vi "LINC Register COSMOS File.vi"(6 "scaling (T)":bool=TRUE, 8 "error in (no error)":errorcluster, 9 "target name override":string, 10 "path":path=path "C:/Projects/LabVIEW 8.5.1 Programs/Common Components/LINC/Examples/APP_TLM.txt", 11 "LINC session":refnum<class "LINC.lvclass">) -> (0 "error out":errorcluster, 3 "dup LINC session":refnum<class "LINC.lvclass">)   [LabVIEW 2018, in "STEPkgDriver_LINC.lvlib" / "LINC.lvclass"]
uses:
  LINC.lvclass
  LINC Format Prototype.ctl
  STEPkgDriver_LINC.lvlib
  LINC Packet.ctl
  LINC Packet Fields.ctl
  LINC Macro.ctl
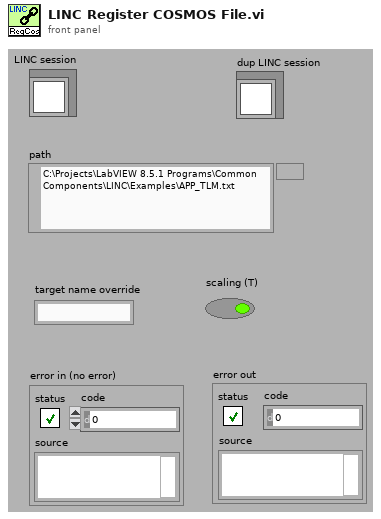
[diagram p1: front panel]
types:
  T1 = typedef "STEPkgDriver_LINC.lvlib/LINC Packet.ctl" = cluster{"type":enum16{"CMD", "TLM"}, "description":string, "hazardous":bool, "item names":string[], "item formats":T2[]}
  T2 = typedef "STEPkgDriver_LINC.lvlib/LINC Format Prototype.ctl" = cluster{"type":string, "bit offset":i32, "bit size":i32, "format":string, "unit":string, "description":string, "state values":i64[], "states":string[], "max":string, "min":string, "default":string, "array":bool, "bit element size":i32, "poly bound":dbl[], "poly scale":cluster{"coefficients":dbl[]}[], "labview size":i32, "simulate":bool, "ID":bool, "required":bool}
  T3 = typedef "STEPkgDriver_LINC.lvlib/LINC Macro.ctl" = cluster{"enabled":bool, "start":i32, "length":i32, "format":string}
  T4 = enum16{"Default", "COMMAND", "SELECT_COMMAND", "HIDDEN", "DISABLED", "DISABLE_MESSAGES", "META", "HAZARDOUS", "PARAMETER", "APPEND_PARAMETER", "ID_PARAMETER", "APPEND_ID_PARAMETER", "ARRAY_PARAMETER", "APPEND_ARRAY_PARAMETER", "SELECT_PARAMETER", "MACRO_APPEND_START", "MACRO_APPEND_END", "PROCESSOR", "ALLOW_SHORT", "STATE", "REQUIRED", "WRITE_CONVERSION", "READ_CONVERSION", "POLY_WRITE_CONVERSION", "POLY_READ_CONVERSION", "SEG_POLY_WRITE_CONVERSION", "SEG_POLY_READ_CONVERSION", "GENERIC_WRITE_CONVERSION_START", "GENERIC_WRITE_CONVERSION_END", "GENERIC_READ_CONVERSION_START", "GENERIC_READ_CONVERSION_END", "FORMAT_STRING ", "MINIMUM_VALUE", "MAXIMUM_VALUE", "DEFAULT_VALUE", "DESCRIPTION", "TELEMETRY", "SELECT_TELEMETRY", "LIMITS_GROUP", "LIMITS_GROUP_ITEM", "ITEM", "APPEND_ITEM", "ID_ITEM", "APPEND_ID_ITEM", "ARRAY_ITEM", "APPEND_ARRAY_ITEM", "LIMITS", "LIMITS_RESPONSE", "UNITS", "SELECT_ITEM"}
  T5 = typedef "STEPkgDriver_LINC.lvlib/LINC Packet Fields.ctl" = cluster{"name":string, "bit offset":string, "bit size":string, "type":string, "min":string, "max":string, "default":string, "description":string, "total size":string}
  T6 = enum16{"state", "required", "poly scale", "format string", "minimum value", "maximum value", "default value", "description", "units"}
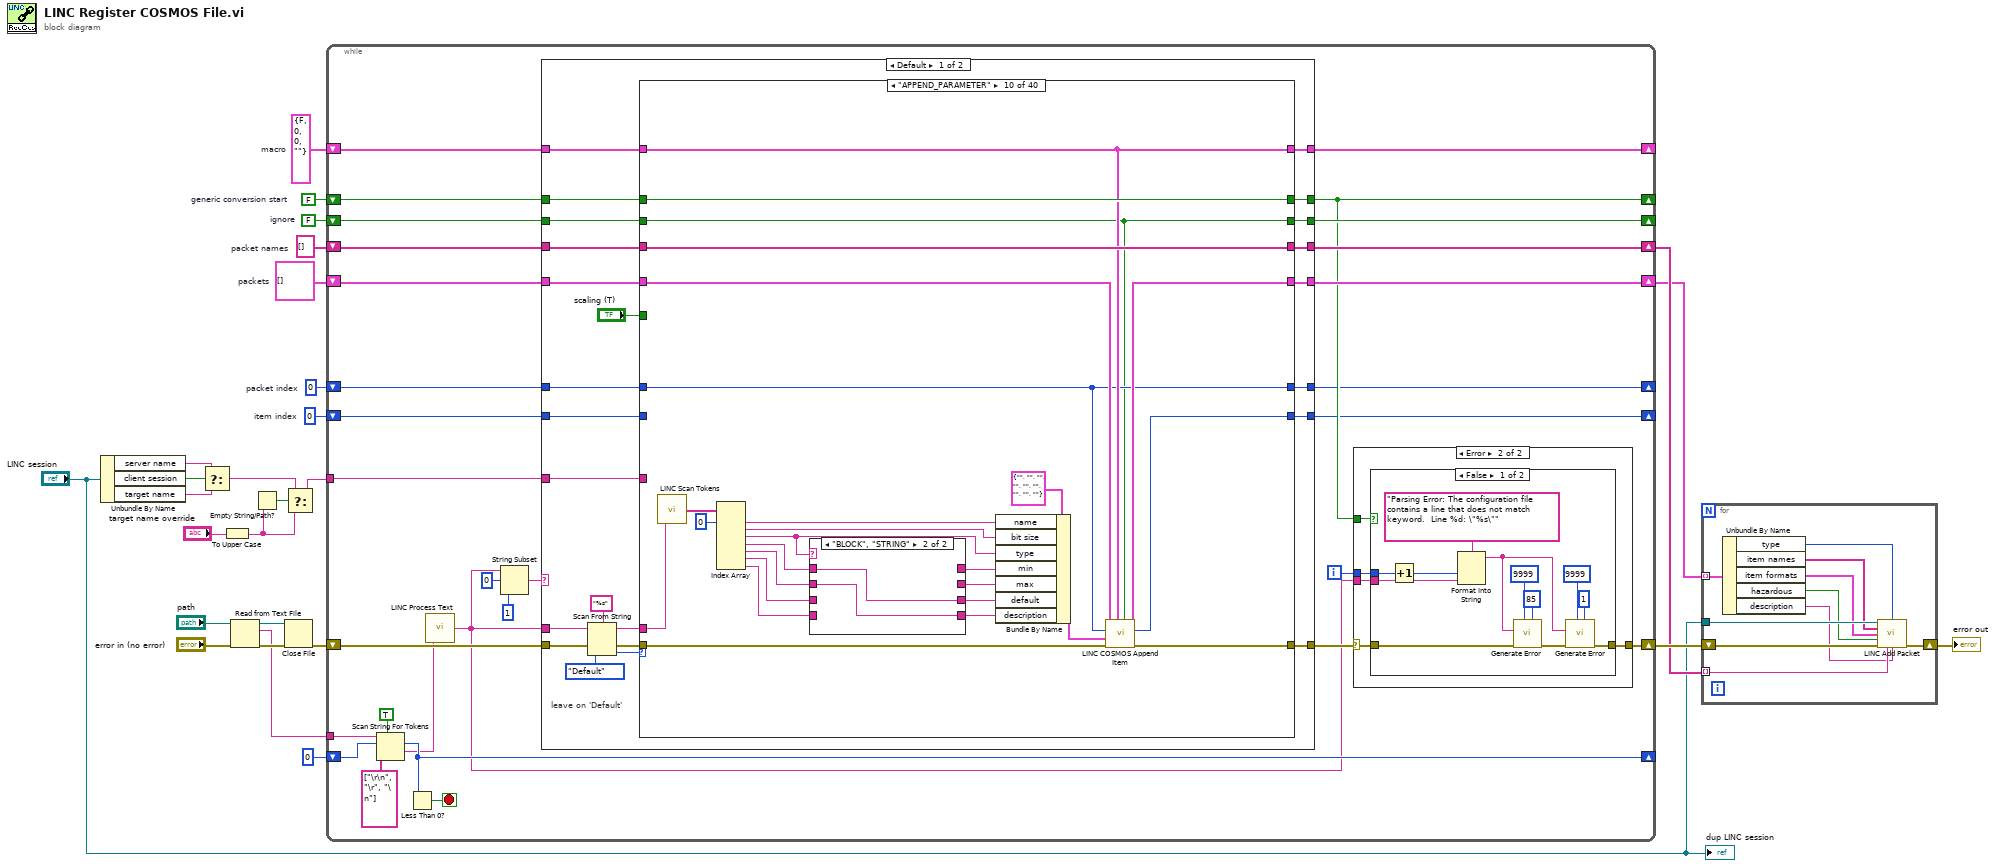
[diagram p0: block diagram]
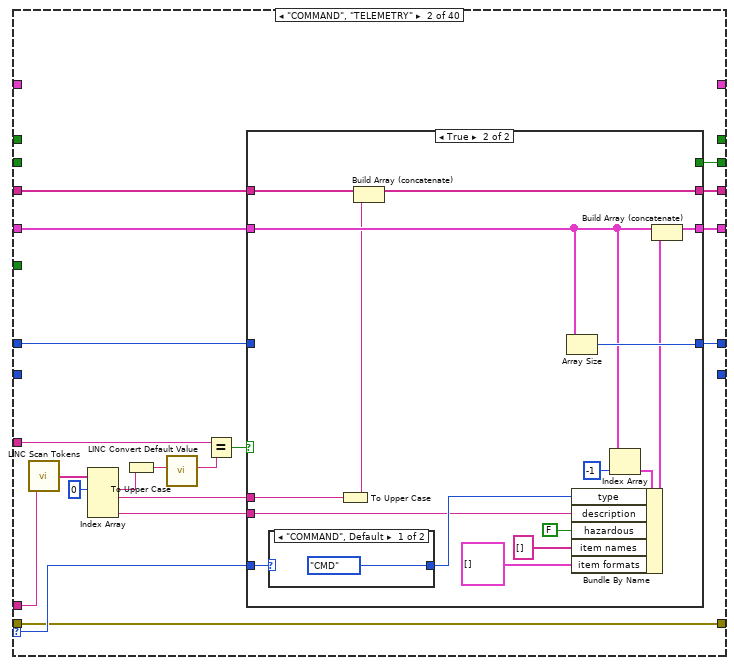
[diagram p5: hidden frame]
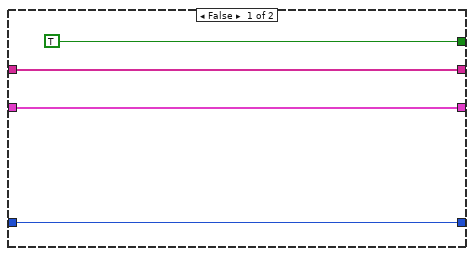
[diagram p6: hidden frame]
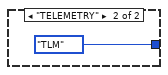
[diagram p7: hidden frame]
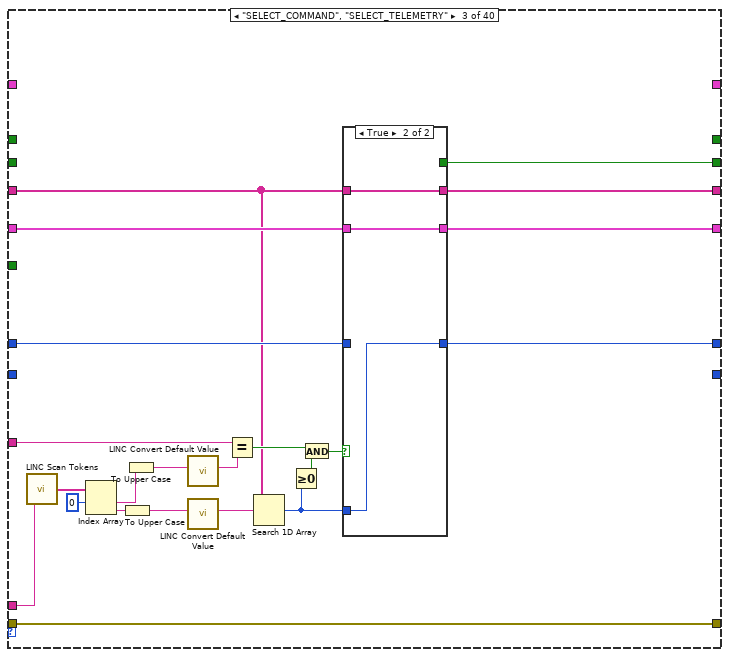
[diagram p8: hidden frame]
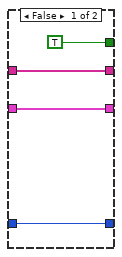
[diagram p9: hidden frame]
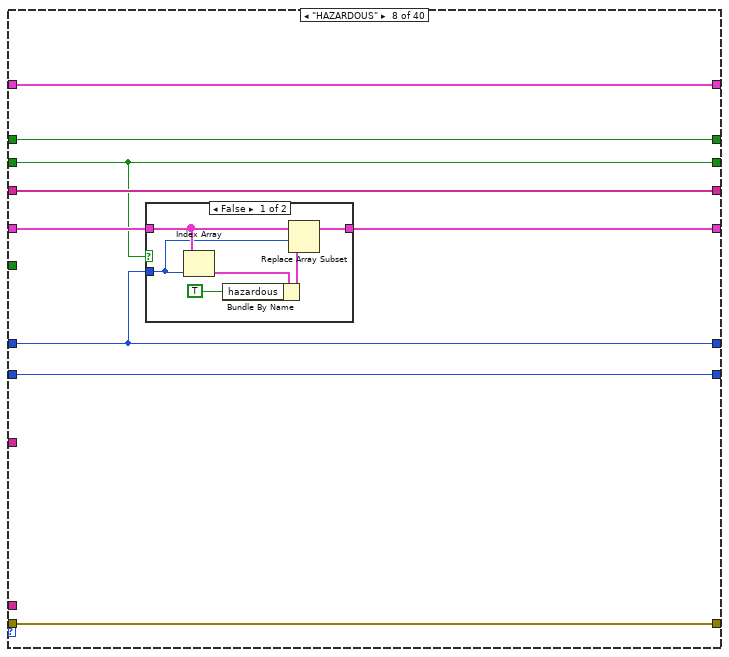
[diagram p14: hidden frame]
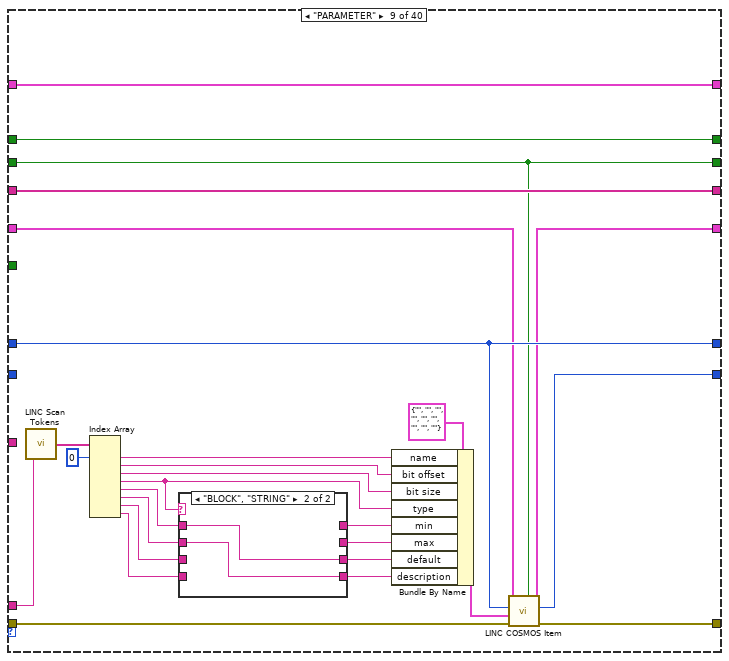
[diagram p16: hidden frame]
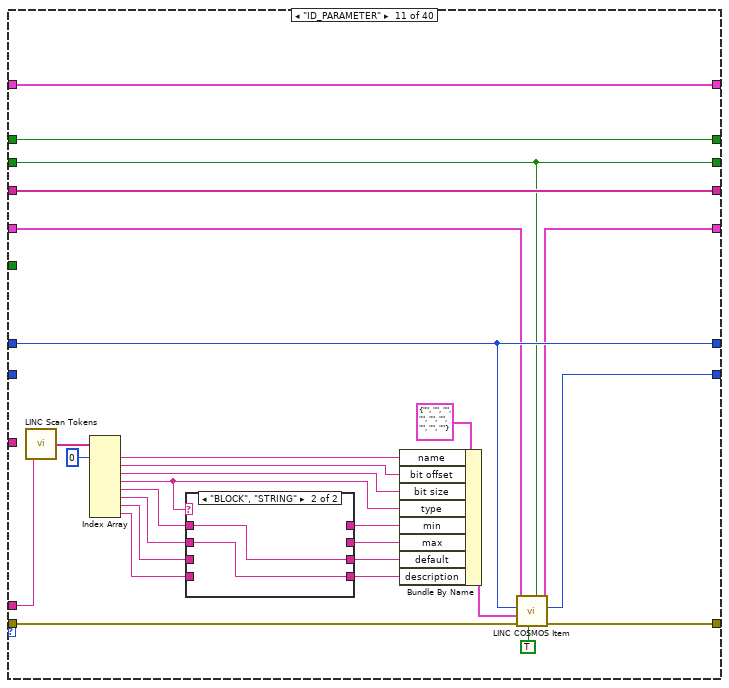
[diagram p19: hidden frame]
diagram:
  w14 = T1[] []  # packets
  w15 = T3 {"enabled"=FALSE, "start"=0, "length"=0, "format"=""}  # macro
  w16 = string[] []  # packet names
  w17 = 0  # item index
  w18 = 0  # packet index
  w19 = FALSE  # generic conversion start
  w22 = FALSE  # ignore
  n1 = Unbundle By Name("LINC session") -> ("server name"=w8:string, "client session"=w9:bool, "target name"=w7:string)
  n2 = Select(t=w8, s=w9, f=w7) -> (s? t:f=w4:string)
  n3 = To Upper Case(1:"target name override") -> (0:w1:string)
  n4 = Read from Text File(file (use dialog)="path", error in="error in (no error)") -> (refnum out=w25:refnum<file>, text=w23:string, error out=w26:errorcluster)  [unwired: 2 in, 1 out]
  n5 = Empty String/Path?(string/path=w1) -> (empty?=w5:bool)
  n6 = Close File(refnum=w25, error in=w26) -> (error out=w21:errorcluster)  [unwired: 1 out]
  n7 = Select(t=w4, s=w5, f=w1) -> (s? t:f=w3:string)
  n8 = while {
    tunnel: w23 -> [w57]
    shift-right: [w53] -> _
    shift-left: 0 -> [w56]
    shift-right: [w37] -> w13
    shift-left: w21 -> [w51]
    shift-right: [w48] -> _
    shift-left: w22 -> [w49]
    shift-right: [w45] -> w11
    shift-left: w16 -> [w47]
    shift-right: [w44] -> w10
    shift-left: w14 -> [w46]
    shift-right: [w39] -> _
    shift-left: w19 -> [w40]
    shift-right: [w32] -> _
    shift-left: w18 -> [w34]
    shift-right: [w31] -> _
    shift-left: w17 -> [w33]
    shift-right: [w29] -> _
    shift-left: w15 -> [w30]
    tunnel: w3 -> [w28]
    i -> [w36]
    stop <- w52 stop-if-true
    n9 = Scan String For Tokens(5:TRUE ("allow empty tokens? (F)"), 6:string[] ["\r\n", "\r", "\n"] ("delimiters (\\s,\\t,\\r,\\n)"), 8:w56, 9:w57) -> (1:w50:string, 2:w53:i32)  [unwired: 2 in, 2 out]
    n10 = Less Than 0?(x=w53) -> (x < 0?=w52:bool)
    n11 = call "LINC Process Text.vi"("line in"=w50) -> ("line out"=w35:string)
    n12 = String Subset(string=w35, offset (0)=0, length (rest)=1 ("length (rest)")) -> (substring=w41:string)
    n13 = case shown="Default" w41 {
      tunnel: w51 -> [w99 w850]
      tunnel: [w93 w850] -> w38
      tunnel: w35 -> [w97 _]
      tunnel: w49 -> [w92 w849]
      tunnel: [w91 w849] -> w48
      tunnel: w47 -> [w90 w848]
      tunnel: w46 -> [w89 w847]
      tunnel: [w88 w848] -> w45
      tunnel: [w87 w847] -> w44
      tunnel: w40 -> [w86 w846]
      tunnel: [w85 w846] -> w39
      tunnel: w34 -> [w84 w845]
      tunnel: w33 -> [w83 w844]
      tunnel: [w82 w845] -> w32
      tunnel: [w81 w844] -> w31
      tunnel: w30 -> [w80 w843]
      tunnel: [w79 w843] -> w29
      tunnel: w28 -> [w77 _]
      frame Default {
        # "leave on 'Default'"
        n14 = Scan From String(format string="%s", input string=w97, error in=w99, default 1=T4."Default") -> (remaining string=w94:string, error out=w96:errorcluster, output 1=w95:T4)  [unwired: 1 in, 1 out]
        n15 = case shown="\"APPEND_PARAMETER\"" w95 {
          selector: w95 -> [_ w125 _ _ _ _ _ _ _ _ _ _ _ _ _ _ _ _ _ _ _ _ _ _ _ _ _ _ _ _ _ _ _ _ _ _ _ _ _ _]
          tunnel: w96 -> [w103 w120 w170 w182 w190 w198 w206 w217 w246 w279 w312 w346 w373 w394 w408 w429 w444 w449 w457 w477 w493 w500 w521 w571 w609 w617 w630 w648 w666 w684 w702 w715 w723 w745 w760 w786 w803 w813 w821 w834]
          tunnel: w94 -> [_ w122 w166 _ _ _ _ _ w249 w280 w315 w347 w375 w396 w403 w430 _ _ _ w484 _ _ w513 w563 _ _ w634 w652 w670 w688 w706 _ _ w732 w761 w772 w804 _ _ w838]
          tunnel: [w103 w120 w170 w182 w190 w198 w206 w217 w245 w278 w311 w345 w372 w393 w408 w429 w444 w449 w457 w476 w492 w500 w520 w570 w609 w617 w629 w647 w665 w683 w701 w715 w723 w744 w759 w785 w802 w813 w821 w833] -> w93
          tunnel: w92 -> [w107 _ _ w185 w193 w201 w209 w210 w235 w268 w300 w334 w358 w379 w410 w423 w442 w452 w460 w463 w485 w503 w514 w564 w612 w620 w623 w641 w659 w677 w695 w718 w726 w729 w747 w768 w790 w816 w824 w827]
          tunnel: [w107 w126 w150 w185 w193 w201 w209 w210 w235 w268 w300 w334 w358 w379 w410 w423 w442 w452 w460 w463 w485 w503 w508 w558 w612 w620 w623 w641 w659 w677 w695 w718 w726 w729 w747 w768 w790 w816 w824 w827] -> w91
          tunnel: w90 -> [w106 w115 w153 w184 w192 w200 w208 w218 w248 w283 w314 w350 w369 w390 w406 w422 w441 w451 w459 w480 w495 w502 w507 w557 w611 w619 w638 w656 w674 w692 w710 w717 w725 w740 w764 w781 w807 w815 w823 w842]
          tunnel: w89 -> [w105 w117 w154 w183 w191 w199 w207 w213 w238 w277 w304 w344 w371 w392 w409 w421 w440 w450 w458 w482 w491 w501 w517 w567 w610 w618 w628 w646 w664 w682 w700 w716 w724 w743 w758 w784 w801 w814 w822 w832]
          tunnel: [w106 w114 w152 w184 w192 w200 w208 w218 w248 w283 w314 w350 w369 w390 w406 w422 w441 w451 w459 w480 w495 w502 w506 w556 w611 w619 w638 w656 w674 w692 w710 w717 w725 w740 w764 w781 w807 w815 w823 w842] -> w88
          tunnel: [w105 w116 w151 w183 w191 w199 w207 w212 w237 w276 w303 w343 w370 w391 w409 w421 w440 w450 w458 w483 w490 w501 w516 w566 w610 w618 w627 w645 w663 w681 w699 w716 w724 w742 w757 w783 w800 w814 w822 w831] -> w87
          tunnel: w86 -> [w104 _ _ w181 w189 w197 w205 w216 w252 w284 w318 w351 w378 w398 w407 w424 w443 w448 w456 w481 w494 w499 w510 w560 _ _ w637 w655 w673 w691 w709 w714 w722 w746 w765 w787 w808 w812 w820 w841]
          tunnel: [w104 _ _ w181 w189 w197 w205 w216 w252 w284 w318 w351 w378 w398 w407 w424 w443 w448 w456 w481 w494 w499 w509 w559 TRUE FALSE w637 w655 w673 w691 w709 w714 w722 w746 w765 w787 w808 w812 w820 w841] -> w85
          tunnel: w84 -> [w102 w108 w156 w179 w187 w195 w203 w211 w239 w269 w305 w335 w368 w389 w400 w420 w439 w446 w454 w479 w488 w497 w519 w569 w607 w615 w626 w644 w662 w680 w698 w712 w720 w730 w749 w769 w792 w810 w818 w830]
          tunnel: w83 -> [w101 _ _ w178 w186 w194 w202 w214 _ _ _ _ _ _ _ w419 w438 w445 w453 w478 w487 w496 w518 w568 w606 w614 w625 w643 w661 w679 w697 w711 w719 _ _ _ _ w809 w817 w829]
          tunnel: [w102 w119 w155 w179 w187 w195 w203 w211 w239 w269 w305 w335 w368 w389 w400 w420 w439 w446 w454 w479 w488 w497 w505 w555 w607 w615 w626 w644 w662 w680 w698 w712 w720 w730 w749 w769 w792 w810 w818 w830] -> w82
          tunnel: [w101 _ _ w178 w186 w194 w202 w214 w236 w275 w302 w342 w367 w388 w399 w419 w438 w445 w453 w478 w487 w496 w504 w554 w606 w614 w625 w643 w661 w679 w697 w711 w719 w739 w756 w780 w799 w809 w817 w829] -> w81
          tunnel: w80 -> [w100 _ _ w180 w188 w196 w204 w215 w247 w270 w313 w337 w374 w395 w401 w426 w437 w447 w455 w475 w489 w498 w515 w565 w608 w616 w624 w642 w660 w678 w696 w713 w721 w741 w750 w782 w793 w811 w819 w828]
          tunnel: [w100 _ _ w180 w188 w196 w204 w215 w247 w270 w313 w337 w374 w395 w401 w425 w436 w447 w455 w475 w489 w498 w511 w561 w608 w616 w624 w642 w660 w678 w696 w713 w721 w741 w750 w782 w793 w811 w819 w828] -> w79
          tunnel: w77 -> [_ w110 w160 _ _ _ _ _ _ _ _ _ _ _ _ _ _ _ _ _ _ _ _ _ _ _ _ _ _ _ _ _ _ _ _ _ _ _ _ _]
          tunnel: "scaling (T)" -> [_ _ _ _ _ _ _ _ _ _ _ _ _ _ _ _ _ _ _ _ _ _ w512 w562 _ _ _ _ _ _ _ _ _ _ _ _ _ _ _ _]
          frame "Default" {
          }
          frame "COMMAND", "TELEMETRY" {
            n16 = call "LINC Scan Tokens.vi"("string"=w122) -> ("tokens"=w124:string[])
            n17 = Index Array(array=w124, index #1=0 ("index")) -> (element #1=w113:string, element #2=w121:string, element #4=w118:string)  [unwired: 3 in, 1 out]
            n18 = To Upper Case(1:w113) -> (0:w112:string)
            n19 = call "LINC Convert Default Value.vi"("default in"=w112) -> ("default out"=w111:string)  [unwired: 10 in]
            n20 = Equal?(x=w110, y=w111) -> (x = y?=w109:bool)
            n21 = case shown="True" w109 {
              tunnel: [TRUE _] -> w126
              tunnel: w125 -> [_ w146]
              tunnel: w121 -> [_ w145]
              tunnel: [w127 w144] -> w119
              tunnel: w118 -> [_ w140]
              tunnel: w117 -> [w128 w136]
              tunnel: [w128 w135] -> w116
              tunnel: w115 -> [w129 w133]
              tunnel: [w129 w132] -> w114
              tunnel: w108 -> [w127 _]
              frame False {
              }
              frame True {
                n22 = case shown="\"COMMAND\", Default" w146 {
                  tunnel: [enum16{"CMD", "TLM"}."CMD" enum16{"CMD", "TLM"}."TLM"] -> w141
                  frame "COMMAND", Default {
                  }
                  frame "TELEMETRY" {
                  }
                }
                n23 = To Upper Case(1:w145) -> (0:w131:string)
                n24 = Build Array (concatenate)(w133, w131) -> (w132:string[])
                n25 = Array Size(array=w136) -> (size(s)=w144:i32)
                n26 = Index Array(array=w136, index=-1) -> (element=w142:T1)
                n27 = Bundle By Name(cluster=w142, "type"=w141, "description"=w140, "hazardous"=FALSE, "item names"=string[] [], "item formats"=T2[] []) -> (w134:T1)
                n28 = Build Array (concatenate)(w136, w134) -> (w135:T1[])
              }
            }
          }
          frame "SELECT_COMMAND", "SELECT_TELEMETRY" {
            n29 = call "LINC Scan Tokens.vi"("string"=w166) -> ("tokens"=w169:string[])
            n30 = Index Array(array=w169, index #1=0 ("index")) -> (element #1=w163:string, element #2=w167:string)  [unwired: 1 in]
            n31 = To Upper Case(1:w167) -> (0:w162:string)
            n32 = To Upper Case(1:w163) -> (0:w165:string)
            n33 = call "LINC Convert Default Value.vi"("default in"=w165) -> ("default out"=w164:string)  [unwired: 10 in]
            n34 = call "LINC Convert Default Value.vi"("default in"=w162) -> ("default out"=w161:string)  [unwired: 10 in]
            n35 = Equal?(x=w160, y=w164) -> (x = y?=w159:bool)
            n36 = Search 1D Array(1D array=w153, element=w161) -> (index of element=w149:i32)  [unwired: 1 in]
            n37 = Greater Or Equal To 0?(x=w149) -> (x >= 0?=w158:bool)
            n38 = And(x=w159, y=w158) -> (x .and. y?=w157:bool)
            n39 = case shown="True" w157 {
              tunnel: w156 -> [w171 _]
              tunnel: w149 -> [_ w177]
              tunnel: [w171 w177] -> w155
              tunnel: w154 -> [w172 w175]
              tunnel: w153 -> [w173 w176]
              tunnel: [w173 w176] -> w152
              tunnel: [w172 w175] -> w151
              tunnel: [TRUE _] -> w150
              frame False {
              }
              frame True {
              }
            }
          }
          frame "HIDDEN" {
            # "Ignore"
          }
          frame "DISABLED" {
            # "Ignore"
          }
          frame "DISABLE_MESSAGES" {
            # "Ignore"
          }
          frame "META" {
            # "Ignore"
          }
          frame "HAZARDOUS" {
            n40 = case shown="False" w210 {
              tunnel: w213 -> [w222 w225]
              tunnel: [w221 w225] -> w212
              tunnel: w211 -> [w220 _]
              frame False {
                n41 = Index Array(array=w222, index=w220) -> (element=w224:T1)
                n42 = Bundle By Name(cluster=w224, "hazardous"=TRUE) -> (w223:T1)
                n43 = Replace Array Subset(array=w222, new element=w223, index=w220) -> (w221:T1[])
              }
              frame True {
              }
            }
          }
          frame "PARAMETER" {
            n44 = call "LINC Scan Tokens.vi"("string"=w249) -> ("tokens"=w251:string[])
            n45 = Index Array(array=w251, index #1=0 ("index")) -> (element #1=w243:string, element #2=w242:string, element #3=w241:string, element #4=w234:string, element #5=w233:string, element #6=w232:string, element #7=w231:string, element #8=w230:string)  [unwired: 7 in]
            n46 = case shown="\"BLOCK\", \"STRING\"" w234 {
              tunnel: [w256 _] -> w229
              tunnel: [w255 _] -> w228
              tunnel: [w254 w258] -> w227
              tunnel: w233 -> [w256 w258]
              tunnel: w232 -> [w255 w257]
              tunnel: w231 -> [w254 _]
              tunnel: w230 -> [w253 _]
              tunnel: [w253 w257] -> w226
              frame Default {
              }
              frame "BLOCK", "STRING" {
              }
            }
            n47 = Bundle By Name(cluster=T5 {"name"="", "bit offset"="", "bit size"="", "type"="", "min"="", "max"="", "default"="", "description"="", "total size"=""} ("packet fields"), "name"=w243, "bit offset"=w242, "bit size"=w241, "type"=w234, "min"=w229, "max"=w228, "default"=w227, "description"=w226) -> (w240:T5)
            n48 = call "LINC COSMOS Item.vi"("ignore"=w235, "error in (no error)"=w246, "packet fields"=w240, "packet index"=w239, "packets in"=w238) -> ("error out"=w245:errorcluster, "item index"=w236:i32, "packets out"=w237:T1[])  [unwired: 4 in]
          }
          frame "APPEND_PARAMETER" {
            n49 = call "LINC Scan Tokens.vi"("string"=w280) -> ("tokens"=w281:string[])
            n50 = Index Array(array=w281, index #1=0 ("index")) -> (element #1=w273:string, element #2=w272:string, element #3=w263:string, element #4=w262:string, element #5=w261:string, element #6=w260:string, element #7=w259:string)  [unwired: 6 in]
            n51 = case shown="\"BLOCK\", \"STRING\"" w263 {
              tunnel: [w288 _] -> w267
              tunnel: [w287 _] -> w266
              tunnel: [w286 w290] -> w265
              tunnel: w262 -> [w288 w290]
              tunnel: w261 -> [w287 w289]
              tunnel: w260 -> [w286 _]
              tunnel: w259 -> [w285 _]
              tunnel: [w285 w289] -> w264
              frame Default {
              }
              frame "BLOCK", "STRING" {
              }
            }
            n52 = Bundle By Name(cluster=T5 {"name"="", "bit offset"="", "bit size"="", "type"="", "min"="", "max"="", "default"="", "description"="", "total size"=""} ("packet fields"), "name"=w273, "bit size"=w272, "type"=w263, "min"=w267, "max"=w266, "default"=w265, "description"=w264) -> (w271:T5)
            n53 = call "LINC COSMOS Append Item.vi"("ignore"=w268, "macro"=w270, "error in (no error)"=w279, "packet fields"=w271, "packet index"=w269, "packets in"=w277) -> ("error out"=w278:errorcluster, "item index"=w275:i32, "packets out"=w276:T1[])  [unwired: 3 in]
          }
          frame "ID_PARAMETER" {
            n54 = call "LINC Scan Tokens.vi"("string"=w315) -> ("tokens"=w317:string[])
            n55 = Index Array(array=w317, index #1=0 ("index")) -> (element #1=w309:string, element #2=w308:string, element #3=w307:string, element #4=w295:string, element #5=w294:string, element #6=w293:string, element #7=w292:string, element #8=w291:string)  [unwired: 7 in]
            n56 = case shown="\"BLOCK\", \"STRING\"" w295 {
              tunnel: [w322 _] -> w299
              tunnel: [w321 _] -> w298
              tunnel: [w320 w324] -> w297
              tunnel: w294 -> [w322 w324]
              tunnel: w293 -> [w321 w323]
              tunnel: w292 -> [w320 _]
              tunnel: w291 -> [w319 _]
              tunnel: [w319 w323] -> w296
              frame Default {
              }
              frame "BLOCK", "STRING" {
              }
            }
            n57 = Bundle By Name(cluster=T5 {"name"="", "bit offset"="", "bit size"="", "type"="", "min"="", "max"="", "default"="", "description"="", "total size"=""} ("packet fields"), "name"=w309, "bit offset"=w308, "bit size"=w307, "type"=w295, "min"=w299, "max"=w298, "default"=w297, "description"=w296) -> (w306:T5)
            n58 = call "LINC COSMOS Item.vi"("ignore"=w300, "ID?"=TRUE, "error in (no error)"=w312, "packet fields"=w306, "packet index"=w305, "packets in"=w304) -> ("error out"=w311:errorcluster, "item index"=w302:i32, "packets out"=w303:T1[])  [unwired: 3 in]
          }
          frame "APPEND_ID_PARAMETER" {
            n59 = call "LINC Scan Tokens.vi"("string"=w347) -> ("tokens"=w348:string[])
            n60 = Index Array(array=w348, index #1=0 ("index")) -> (element #1=w340:string, element #2=w339:string, element #3=w332:string, element #4=w328:string, element #5=w327:string, element #6=w326:string, element #7=w325:string)  [unwired: 6 in]
            n61 = case shown="\"BLOCK\", \"STRING\"" w332 {
              tunnel: [w355 _] -> w333
              tunnel: [w354 _] -> w331
              tunnel: [w353 w357] -> w330
              tunnel: w328 -> [w355 w357]
              tunnel: w327 -> [w354 w356]
              tunnel: w326 -> [w353 _]
              tunnel: w325 -> [w352 _]
              tunnel: [w352 w356] -> w329
              frame Default {
              }
              frame "BLOCK", "STRING" {
              }
            }
            n62 = Bundle By Name(cluster=T5 {"name"="", "bit offset"="", "bit size"="", "type"="", "min"="", "max"="", "default"="", "description"="", "total size"=""} ("packet fields"), "name"=w340, "bit size"=w339, "type"=w332, "min"=w333, "max"=w331, "default"=w330, "description"=w329) -> (w338:T5)
            n63 = call "LINC COSMOS Append Item.vi"("ignore"=w334, "ID?"=TRUE, "macro"=w337, "error in (no error)"=w346, "packet fields"=w338, "packet index"=w335, "packets in"=w344) -> ("error out"=w345:errorcluster, "item index"=w342:i32, "packets out"=w343:T1[])  [unwired: 2 in]
          }
          frame "ARRAY_PARAMETER", "ARRAY_ITEM" {
            n64 = call "LINC Scan Tokens.vi"("string"=w375) -> ("tokens"=w377:string[])
            n65 = Index Array(array=w377, index #1=0 ("index")) -> (element #1=w365:string, element #2=w364:string, element #3=w363:string, element #4=w362:string, element #5=w360:string, element #6=w359:string)  [unwired: 5 in]
            n66 = Bundle By Name(cluster=T5 {"name"="", "bit offset"="", "bit size"="", "type"="", "min"="", "max"="", "default"="", "description"="", "total size"=""} ("packet fields"), "name"=w365, "bit offset"=w364, "bit size"=w363, "type"=w362, "total size"=w360, "description"=w359) -> (w361:T5)
            n67 = call "LINC COSMOS Array Item.vi"("ignore"=w358, "error in (no error)"=w373, "packet fields"=w361, "packet index"=w368, "packets in"=w371) -> ("error out"=w372:errorcluster, "item index"=w367:i32, "packets out"=w370:T1[])  [unwired: 4 in]
          }
          frame "APPEND_ARRAY_PARAMETER", "APPEND_ARRAY_ITEM" {
            n68 = call "LINC Scan Tokens.vi"("string"=w396) -> ("tokens"=w397:string[])
            n69 = Index Array(array=w397, index #1=0 ("index")) -> (element #1=w381:string, element #2=w386:string, element #3=w385:string, element #4=w383:string, element #5=w382:string)  [unwired: 4 in]
            n70 = Bundle By Name(cluster=T5 {"name"="", "bit offset"="", "bit size"="", "type"="", "min"="", "max"="", "default"="", "description"="", "total size"=""} ("packet fields"), "name"=w381, "bit size"=w386, "type"=w385, "total size"=w383, "description"=w382) -> (w384:T5)
            n71 = call "LINC COSMOS Append Array Item.vi"("ignore"=w379, "error in (no error)"=w394, "packet fields"=w384, "packet index"=w389, "packets in"=w392) -> ("error out"=w393:errorcluster, "item index"=w388:i32, "packets out"=w391:T1[])  [unwired: 4 in]
          }
          frame "SELECT_PARAMETER", "SELECT_ITEM" {
            n72 = call "LINC Scan Tokens.vi"("string"=w403) -> ("tokens"=w405:string[])
            n73 = Index Array(array=w405, index=0) -> (element=w402:string)
            n74 = Search 1D Array(1D array=w406, element=w402) -> (index of element=w399:i32)  [unwired: 1 in]
          }
          frame "MACRO_APPEND_START" {
            n75 = call "LINC Scan Tokens.vi"("string"=w430) -> ("tokens"=w432:string[])
            n76 = Index Array(array=w432, index #1=0 ("index")) -> (element #1=w428:string, element #2=w427:string, element #3=w413:string)  [unwired: 2 in]
            n77 = Empty String/Path?(string/path=w413) -> (empty?=w414:bool)
            n78 = case shown="True" w414 {
              tunnel: w413 -> [w433 _]
              tunnel: [w433 "%s%d"] -> w412
              frame False {
              }
              frame True {
              }
            }
            n79 = Decimal String To Number(string=w428) -> (number=w417:i32)  [unwired: 2 in, 1 out]
            n80 = Decimal String To Number(string=w427) -> (number=w418:i32)  [unwired: 2 in, 1 out]
            n81 = Subtract(x=w418, y=w417) -> (x-y=w416:i32)
            n82 = Increment(x=w416) -> (x+1=w415:i32)
            n83 = Bundle By Name(cluster=w426, "enabled"=TRUE, "start"=w417, "length"=w415, "format"=w412) -> (w425:T3)
          }
          frame "MACRO_APPEND_END" {
            n84 = Bundle By Name(cluster=w437, "enabled"=FALSE) -> (w436:T3)
          }
          frame "PROCESSOR" {
            # "Ignore"
          }
          frame "ALLOW_SHORT" {
            # "Ignore"
          }
          frame "STATE" {
            n85 = call "LINC Scan Tokens.vi"("string"=w484) -> ("tokens"=w473:string[])
            n86 = Index Array(array=w473, index #1=0 ("index")) -> (element #1=w471:string, element #2=w472:string)  [unwired: 1 in]
            n87 = Decimal String To Number(string=w472, default (0L)=i64 0) -> (number=w468:i64)  [unwired: 1 in, 1 out]
            n88 = To Upper Case(1:w471) -> (0:w462:string)
            n89 = call "LINC Convert Default Value.vi"("default in"=w462) -> ("default out"=w461:string)  [unwired: 10 in]
            n90 = Build Array(w461) -> (w466:string[])
            n91 = Build Array(w468) -> (w465:i64[])
            n92 = Bundle By Name(cluster=T2 {"type"="", "bit offset"=0, "bit size"=0, "format"="", "unit"="", "description"="", "state values"=[], "states"=[], "max"="", "min"="", "default"="", "array"=FALSE, "bit element size"=0, "poly bound"=[], "poly scale"=[], "labview size"=0, "simulate"=FALSE, "ID"=FALSE, "required"=FALSE} ("item"), "states"=w466, "state values"=w465) -> (w464:T2)
            n93 = call "LINC COSMOS Update Item.vi"("property"=T6."state", "ignore"=w463, "item"=w464, "macro"=w475, "error in (no error)"=w477, "item index"=w478, "packet index"=w479, "packets in"=w482) -> ("error out"=w476:errorcluster, "packets out"=w483:T1[])  [unwired: 2 in]
          }
          frame "REQUIRED" {
            n94 = call "LINC COSMOS Update Item.vi"("property"=T6."required", "ignore"=w485, "macro"=w489, "error in (no error)"=w493, "item index"=w487, "packet index"=w488, "packets in"=w491) -> ("error out"=w492:errorcluster, "packets out"=w490:T1[])  [unwired: 3 in]
          }
          frame "WRITE_CONVERSION", "READ_CONVERSION" {
            # "Ignore.  This modifier points to custom ruby script and cannot be handled."
          }
          frame "POLY_WRITE_CONVERSION", "POLY_READ_CONVERSION" {
            n95 = case shown="True" w512 {
              tunnel: w521 -> [w528 w547]
              tunnel: [w528 w546] -> w520
              tunnel: w519 -> [w523 w531]
              tunnel: w518 -> [w522 w530]
              tunnel: w517 -> [w529 w545]
              tunnel: [w529 w544] -> w516
              tunnel: w515 -> [w527 w535]
              tunnel: w514 -> [w525 w533]
              tunnel: w513 -> [_ w543]
              tunnel: [w527 w535] -> w511
              tunnel: w510 -> [w526 w534]
              tunnel: [w526 w534] -> w509
              tunnel: [w525 w533] -> w508
              tunnel: w507 -> [w524 w532]
              tunnel: [w524 w532] -> w506
              tunnel: [w523 w531] -> w505
              tunnel: [w522 w530] -> w504
              frame False {
              }
              frame True {
                # "We treat a standard polynomial (unsegmented) identically to a segmented polynomial during scaling.  For unsegmented, there will be only one set of coefficients and a single lower bound (poly bound).  The value of poly bound doesn't matter since the scaling will just use the only coefficients available."
                n96 = String Subset(string=w543, offset (0)=1) -> (substring=w541:string)  [unwired: 1 in]
                n97 = Spreadsheet String To Array(delimiter (Tab)=" ", format string="%f", spreadsheet string=w541, array type (2D Dbl)=dbl[] []) -> (array=w540:dbl[])
                n98 = Bundle(w540) -> (w539:cluster{dbl[]})  [unwired: 1 in]
                n99 = Build Array(0.0) -> (w536:dbl[])
                n100 = Build Array(w539) -> (w538:cluster{dbl[]}[])
                n101 = Bundle By Name(cluster=T2 {"type"="", "bit offset"=0, "bit size"=0, "format"="", "unit"="", "description"="", "state values"=[], "states"=[], "max"="", "min"="", "default"="", "array"=FALSE, "bit element size"=0, "poly bound"=[], "poly scale"=[], "labview size"=0, "simulate"=FALSE, "ID"=FALSE, "required"=FALSE} ("item"), "poly bound"=w536, "poly scale"=w538) -> (w548:T2)
                n102 = call "LINC COSMOS Update Item.vi"("property"=T6."poly scale", "ignore"=w533, "item"=w548, "macro"=w535, "error in (no error)"=w547, "item index"=w530, "packet index"=w531, "packets in"=w545) -> ("error out"=w546:errorcluster, "packets out"=w544:T1[])  [unwired: 2 in]
              }
            }
          }
          frame "SEG_POLY_WRITE_CONVERSION", "SEG_POLY_READ_CONVERSION" {
            n103 = case shown="False" w562 {
              tunnel: w571 -> [w578 w599]
              tunnel: [w578 w598] -> w570
              tunnel: w569 -> [w573 w581]
              tunnel: w568 -> [w572 w580]
              tunnel: w567 -> [w579 w597]
              tunnel: [w579 w596] -> w566
              tunnel: w565 -> [w577 w585]
              tunnel: w564 -> [w575 w583]
              tunnel: w563 -> [_ w595]
              tunnel: [w577 w585] -> w561
              tunnel: w560 -> [w576 w584]
              tunnel: [w576 w584] -> w559
              tunnel: [w575 w583] -> w558
              tunnel: w557 -> [w574 w582]
              tunnel: [w574 w582] -> w556
              tunnel: [w573 w581] -> w555
              tunnel: [w572 w580] -> w554
              frame False {
              }
              frame True {
                # "The first value is the lower bound.  Pick it off and set the rest of the values as coefficients."
                n104 = String Subset(string=w595, offset (0)=1) -> (substring=w593:string)  [unwired: 1 in]
                n105 = Spreadsheet String To Array(delimiter (Tab)=" ", format string="%f", spreadsheet string=w593, array type (2D Dbl)=dbl[] []) -> (array=w590:dbl[])
                n106 = Delete From Array(array=w590, index=0) -> (deleted portion=w588:dbl, array with subset deleted=w589:dbl[])  [unwired: 1 in]
                n107 = Bundle(w589) -> (w592:cluster{dbl[]})  [unwired: 1 in]
                n108 = Build Array(w588) -> (w586:dbl[])
                n109 = Build Array(w592) -> (w591:cluster{dbl[]}[])
                n110 = Bundle By Name(cluster=T2 {"type"="", "bit offset"=0, "bit size"=0, "format"="", "unit"="", "description"="", "state values"=[], "states"=[], "max"="", "min"="", "default"="", "array"=FALSE, "bit element size"=0, "poly bound"=[], "poly scale"=[], "labview size"=0, "simulate"=FALSE, "ID"=FALSE, "required"=FALSE} ("item"), "poly scale"=w591, "poly bound"=w586) -> (w600:T2)
                n111 = call "LINC COSMOS Update Item.vi"("property"=T6."poly scale", "ignore"=w583, "item"=w600, "macro"=w585, "error in (no error)"=w599, "item index"=w580, "packet index"=w581, "packets in"=w597) -> ("error out"=w598:errorcluster, "packets out"=w596:T1[])  [unwired: 2 in]
              }
            }
          }
          frame "GENERIC_WRITE_CONVERSION_START", "GENERIC_READ_CONVERSION_START" {
          }
          frame "GENERIC_WRITE_CONVERSION_END", "GENERIC_READ_CONVERSION_END" {
          }
          frame "FORMAT_STRING " {
            n112 = call "LINC Scan Tokens.vi"("string"=w634) -> ("tokens"=w636:string[])
            n113 = Index Array(array=w636, index=0) -> (element=w622:string)
            n114 = Bundle By Name(cluster=T2 {"type"="", "bit offset"=0, "bit size"=0, "format"="", "unit"="", "description"="", "state values"=[], "states"=[], "max"="", "min"="", "default"="", "array"=FALSE, "bit element size"=0, "poly bound"=[], "poly scale"=[], "labview size"=0, "simulate"=FALSE, "ID"=FALSE, "required"=FALSE} ("item"), "format"=w622) -> (w631:T2)
            n115 = call "LINC COSMOS Update Item.vi"("property"=T6."format string", "ignore"=w623, "item"=w631, "macro"=w624, "error in (no error)"=w630, "item index"=w625, "packet index"=w626, "packets in"=w628) -> ("error out"=w629:errorcluster, "packets out"=w627:T1[])  [unwired: 2 in]
          }
          frame "MINIMUM_VALUE" {
            n116 = call "LINC Scan Tokens.vi"("string"=w652) -> ("tokens"=w654:string[])
            n117 = Index Array(array=w654, index=0) -> (element=w640:string)
            n118 = call "LINC Convert Default Value.vi"("default in"=w640) -> ("default out"=w639:string)  [unwired: 10 in]
            n119 = Bundle By Name(cluster=T2 {"type"="", "bit offset"=0, "bit size"=0, "format"="", "unit"="", "description"="", "state values"=[], "states"=[], "max"="", "min"="", "default"="", "array"=FALSE, "bit element size"=0, "poly bound"=[], "poly scale"=[], "labview size"=0, "simulate"=FALSE, "ID"=FALSE, "required"=FALSE} ("item"), "min"=w639) -> (w649:T2)
            n120 = call "LINC COSMOS Update Item.vi"("property"=T6."minimum value", "ignore"=w641, "item"=w649, "macro"=w642, "error in (no error)"=w648, "item index"=w643, "packet index"=w644, "packets in"=w646) -> ("error out"=w647:errorcluster, "packets out"=w645:T1[])  [unwired: 2 in]
          }
          frame "MAXIMUM_VALUE" {
            n121 = call "LINC Scan Tokens.vi"("string"=w670) -> ("tokens"=w672:string[])
            n122 = Index Array(array=w672, index=0) -> (element=w658:string)
            n123 = call "LINC Convert Default Value.vi"("default in"=w658) -> ("default out"=w657:string)  [unwired: 10 in]
            n124 = Bundle By Name(cluster=T2 {"type"="", "bit offset"=0, "bit size"=0, "format"="", "unit"="", "description"="", "state values"=[], "states"=[], "max"="", "min"="", "default"="", "array"=FALSE, "bit element size"=0, "poly bound"=[], "poly scale"=[], "labview size"=0, "simulate"=FALSE, "ID"=FALSE, "required"=FALSE} ("item"), "max"=w657) -> (w667:T2)
            n125 = call "LINC COSMOS Update Item.vi"("property"=T6."maximum value", "ignore"=w659, "item"=w667, "macro"=w660, "error in (no error)"=w666, "item index"=w661, "packet index"=w662, "packets in"=w664) -> ("error out"=w665:errorcluster, "packets out"=w663:T1[])  [unwired: 2 in]
          }
          frame "DEFAULT_VALUE" {
            n126 = call "LINC Scan Tokens.vi"("string"=w688) -> ("tokens"=w690:string[])
            n127 = Index Array(array=w690, index=0) -> (element=w676:string)
            n128 = call "LINC Convert Default Value.vi"("default in"=w676) -> ("default out"=w675:string)  [unwired: 10 in]
            n129 = Bundle By Name(cluster=T2 {"type"="", "bit offset"=0, "bit size"=0, "format"="", "unit"="", "description"="", "state values"=[], "states"=[], "max"="", "min"="", "default"="", "array"=FALSE, "bit element size"=0, "poly bound"=[], "poly scale"=[], "labview size"=0, "simulate"=FALSE, "ID"=FALSE, "required"=FALSE} ("item"), "default"=w675) -> (w685:T2)
            n130 = call "LINC COSMOS Update Item.vi"("property"=T6."default value", "ignore"=w677, "item"=w685, "macro"=w678, "error in (no error)"=w684, "item index"=w679, "packet index"=w680, "packets in"=w682) -> ("error out"=w683:errorcluster, "packets out"=w681:T1[])  [unwired: 2 in]
          }
          frame "DESCRIPTION" {
            n131 = call "LINC Scan Tokens.vi"("string"=w706) -> ("tokens"=w708:string[])
            n132 = Index Array(array=w708, index=0) -> (element=w694:string)
            n133 = call "LINC Convert Default Value.vi"("default in"=w694) -> ("default out"=w693:string)  [unwired: 10 in]
            n134 = Bundle By Name(cluster=T2 {"type"="", "bit offset"=0, "bit size"=0, "format"="", "unit"="", "description"="", "state values"=[], "states"=[], "max"="", "min"="", "default"="", "array"=FALSE, "bit element size"=0, "poly bound"=[], "poly scale"=[], "labview size"=0, "simulate"=FALSE, "ID"=FALSE, "required"=FALSE} ("item"), "description"=w693) -> (w703:T2)
            n135 = call "LINC COSMOS Update Item.vi"("property"=T6."description", "ignore"=w695, "item"=w703, "macro"=w696, "error in (no error)"=w702, "item index"=w697, "packet index"=w698, "packets in"=w700) -> ("error out"=w701:errorcluster, "packets out"=w699:T1[])  [unwired: 2 in]
          }
          frame "LIMITS_GROUP" {
            # "Ignore"
          }
          frame "LIMITS_GROUP_ITEM" {
            # "Ignore"
          }
          frame "ITEM" {
            n136 = call "LINC Scan Tokens.vi"("string"=w732) -> ("tokens"=w738:string[])
            n137 = Index Array(array=w738, index #1=0 ("index")) -> (element #1=w735:string, element #2=w734:string, element #3=w733:string, element #4=w728:string, element #5=w727:string)  [unwired: 4 in]
            n138 = Bundle By Name(cluster=T5 {"name"="", "bit offset"="", "bit size"="", "type"="", "min"="", "max"="", "default"="", "description"="", "total size"=""} ("packet fields"), "name"=w735, "bit offset"=w734, "bit size"=w733, "type"=w728, "description"=w727) -> (w731:T5)
            n139 = call "LINC COSMOS Item.vi"("ignore"=w729, "error in (no error)"=w745, "packet fields"=w731, "packet index"=w730, "packets in"=w743) -> ("error out"=w744:errorcluster, "item index"=w739:i32, "packets out"=w742:T1[])  [unwired: 4 in]
          }
          frame "APPEND_ITEM" {
            n140 = call "LINC Scan Tokens.vi"("string"=w761) -> ("tokens"=w762:string[])
            n141 = Index Array(array=w762, index #1=0 ("index")) -> (element #1=w754:string, element #2=w753:string, element #3=w752:string, element #4=w748:string)  [unwired: 3 in]
            n142 = Bundle By Name(cluster=T5 {"name"="", "bit offset"="", "bit size"="", "type"="", "min"="", "max"="", "default"="", "description"="", "total size"=""} ("packet fields"), "name"=w754, "bit size"=w753, "type"=w752, "description"=w748) -> (w751:T5)
            n143 = call "LINC COSMOS Append Item.vi"("ignore"=w747, "macro"=w750, "error in (no error)"=w760, "packet fields"=w751, "packet index"=w749, "packets in"=w758) -> ("error out"=w759:errorcluster, "item index"=w756:i32, "packets out"=w757:T1[])  [unwired: 3 in]
          }
          frame "ID_ITEM" {
            n144 = call "LINC Scan Tokens.vi"("string"=w772) -> ("tokens"=w779:string[])
            n145 = Index Array(array=w779, index #1=0 ("index")) -> (element #1=w776:string, element #2=w775:string, element #3=w774:string, element #4=w773:string, element #5=w766:string, element #6=w767:string)  [unwired: 5 in]
            n146 = Bundle By Name(cluster=T5 {"name"="", "bit offset"="", "bit size"="", "type"="", "min"="", "max"="", "default"="", "description"="", "total size"=""} ("packet fields"), "name"=w776, "bit offset"=w775, "bit size"=w774, "type"=w773, "default"=w766, "description"=w767) -> (w771:T5)
            n147 = call "LINC COSMOS Item.vi"("ignore"=w768, "ID?"=TRUE, "error in (no error)"=w786, "packet fields"=w771, "packet index"=w769, "packets in"=w784) -> ("error out"=w785:errorcluster, "item index"=w780:i32, "packets out"=w783:T1[])  [unwired: 3 in]
          }
          frame "APPEND_ID_ITEM" {
            n148 = call "LINC Scan Tokens.vi"("string"=w804) -> ("tokens"=w805:string[])
            n149 = Index Array(array=w805, index #1=0 ("index")) -> (element #1=w797:string, element #2=w796:string, element #3=w795:string, element #4=w788:string, element #5=w789:string)  [unwired: 4 in]
            n150 = Bundle By Name(cluster=T5 {"name"="", "bit offset"="", "bit size"="", "type"="", "min"="", "max"="", "default"="", "description"="", "total size"=""} ("packet fields"), "name"=w797, "bit size"=w796, "type"=w795, "default"=w788, "description"=w789) -> (w794:T5)
            n151 = call "LINC COSMOS Append Item.vi"("ignore"=w790, "ID?"=TRUE, "macro"=w793, "error in (no error)"=w803, "packet fields"=w794, "packet index"=w792, "packets in"=w801) -> ("error out"=w802:errorcluster, "item index"=w799:i32, "packets out"=w800:T1[])  [unwired: 2 in]
          }
          frame "LIMITS" {
          }
          frame "LIMITS_RESPONSE" {
            # "Ignore"
          }
          frame "UNITS" {
            n152 = call "LINC Scan Tokens.vi"("string"=w838) -> ("tokens"=w840:string[])
            n153 = Index Array(array=w840, index=0) -> (element=w826:string)
            n154 = call "LINC Convert Default Value.vi"("default in"=w826) -> ("default out"=w825:string)  [unwired: 10 in]
            n155 = Bundle By Name(cluster=T2 {"type"="", "bit offset"=0, "bit size"=0, "format"="", "unit"="", "description"="", "state values"=[], "states"=[], "max"="", "min"="", "default"="", "array"=FALSE, "bit element size"=0, "poly bound"=[], "poly scale"=[], "labview size"=0, "simulate"=FALSE, "ID"=FALSE, "required"=FALSE} ("item"), "unit"=w825) -> (w835:T2)
            n156 = call "LINC COSMOS Update Item.vi"("property"=T6."units", "ignore"=w827, "item"=w835, "macro"=w828, "error in (no error)"=w834, "item index"=w829, "packet index"=w830, "packets in"=w832) -> ("error out"=w833:errorcluster, "packets out"=w831:T1[])  [unwired: 2 in]
          }
        }
      }
      frame "", "#" {
        # "Filter out blank lines and comments"
      }
    }
    n157 = case shown="Error" w38 {
      selector: w38 -> [w58 w62]
      tunnel: w39 -> [_ w63]
      tunnel: [w58 w61] -> w37
      tunnel: w36 -> [_ w60]
      tunnel: w35 -> [_ w59]
      frame No Error {
      }
      frame Error {
        n158 = case shown="False" w63 {
          tunnel: w62 -> [w75 _]
          tunnel: [w65 _] -> w61
          tunnel: w59 -> [w71 _]
          tunnel: w60 -> [w70 _]
          frame False {
            n159 = Increment(x=w70) -> (x+1=w69:i32)
            n160 = Format Into String(format string="Parsing Error: The configuration file contains a line that does not match keyword.  Line %d: \"%s\"" ("description"), w69, w71) -> (resulting string=w64:string)  [unwired: 2 in, 1 out]
            n161 = call "Generate Error.vi"("match code"=85, "error code (-1301)"=9999, "error in"=w75, "description"=w64) -> ("error out"=w66:errorcluster)  [unwired: 7 in]
            n162 = call "Generate Error.vi"("match code"=1, "error code (-1301)"=9999, "error in"=w66, "description"=w64) -> ("error out"=w65:errorcluster)  [unwired: 7 in]
          }
          frame True {
          }
        }
      }
    }
  }
  n163 = for {
    tunnel: "LINC session" -> [w860]
    shift-right: [w858] -> w12
    shift-left: w13 -> [w859]
    tunnel: w11 -> [w857] mode=indexing
    tunnel: w10 -> [w856] mode=indexing
    n164 = Unbundle By Name(w856) -> ("type"=w855:enum16{"CMD", "TLM"}, "item names"=w854:string[], "item formats"=w853:T2[], "hazardous"=w852:bool, "description"=w851:string)
    n165 = call "LINC Add Packet.vi"("LINC session"=w860, "type (CMD)"=w855, "item names in"=w854, "item formats in"=w853, "hazardous"=w852, "e rror in (no error)"=w859, "packet name"=w857, "packet description"=w851) -> ("error out"=w858:errorcluster)  [unwired: 6 in, 1 out]
  }
  "error out" <- w12
  "dup LINC session" <- "LINC session"
